vi "TTA_MATLAB_BDSSig.vi"(0 "Signal Settings":string="TTAData.Signals.BDS", 11 "error in":errorcluster) -> (4 "Success":bool, 15 "error out":errorcluster)   [LabVIEW 2016]
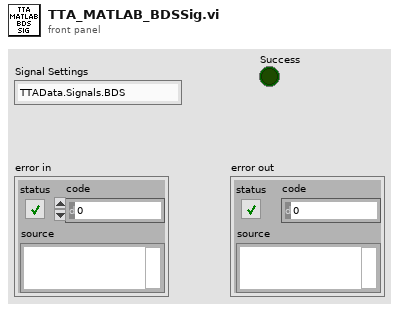
[diagram p1: front panel]
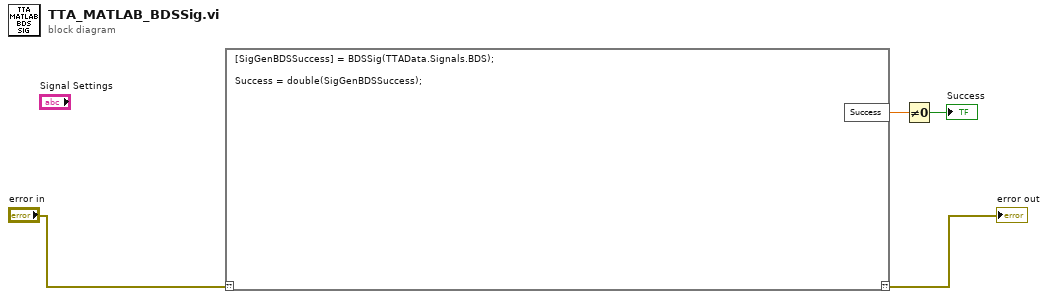
[diagram p0: block diagram]
diagram:
  n1 = script code="[SigGenBDSSuccess] = BDSSig(TTAData.Signals.BDS);\n\nSuccess = double(SigGenBDSSuccess);"("??"="error in") -> ("??"=→"error out":errorcluster, "Success"=w2:dbl)
  n2 = Not Equal To 0?(x=w2) -> (x != 0?=→"Success":bool)
